vi "Actor Core.vi"(8 "error in":errorcluster, 11 "Pulse Controller in":refnum<class "Pulse Controller.lvclass">) -> (0 "error out":errorcluster, 3 "Actor out":refnum<class "Actor.lvclass">)   [LabVIEW 2016, in "Pulse Controller.lvclass"]
doc: "(<B>Filename</B>: Actor Framework.lvlib:Actor.lvclass:Actor Core.vi)\n\nReceives messages to the actor, reacts to them, and initiates any error handling that may shut the actor down.\n\nDescendant classes may override this VI to append parallel tasks for the actor to complete while it handles messages. Overrides use the Call Parent Method node."
uses:
  Pulse Controller.lvclass
  C:/github/LabActor/Template Module/Template Module.lvclass
  C:/Program Files/National Instruments/LabVIEW 2016/vi.lib/ActorFramework/Actor/Actor.lvclass
  <vilib>/ActorFramework/Actor/Actor.lvclass
  Pulse Controller Configuration.ctl
  Template Module/Template Module.lvclass/Template Module.ctl
  <vilib>/ActorFramework/Actor/Actor.lvclass/Actor.ctl
  <vilib>/ActorFramework/Message Enqueuer/Message Enqueuer.lvclass/Message Enqueuer.ctl
  Template Module/Read stop event.vi
  <vilib>/ActorFramework/Message Enqueuer/Init from Existing Queue.vi
  <vilib>/ActorFramework/Message Enqueuer/Enqueue.vi
  Worker Messages/Trigger Msg/Trigger Msg.lvclass
  C:/Program Files/National Instruments/LabVIEW 2016/vi.lib/ActorFramework/Message/Message.lvclass
  <vilib>/ActorFramework/Message Priority Queue/Priority Enqueue.vi
  Process Controller/Process Controller.lvclass
  <vilib>/ActorFramework/Message Enqueuer/Message Enqueuer.lvclass
panel:
  in  "Trigger":bool
  in  "Configuration":T1={"Pre-trigger duration"=-1.0, "Post-trigger duration"=-1.0, "Open plot after pulse"=TRUE} {"Pre-trigger duration" format="%#_6p"; "Post-trigger duration" format="%#_6p"}
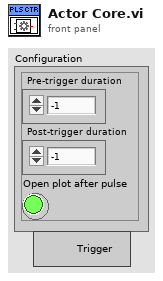
[diagram p1: front panel]
types:
  T1 = typedef "Pulse Controller Configuration.ctl" = cluster{"Pre-trigger duration":dbl, "Post-trigger duration":dbl, "Open plot after pulse":bool}
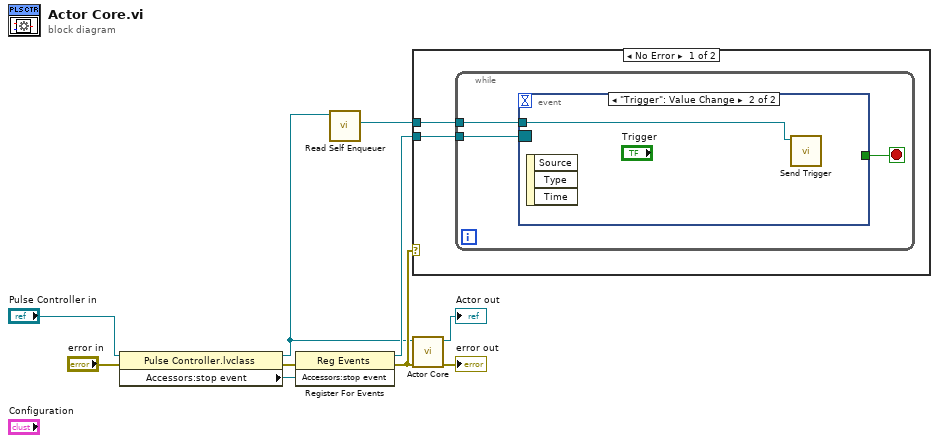
[diagram p0: block diagram]
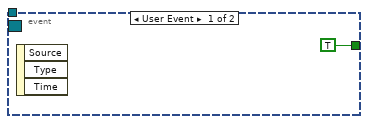
[diagram p2: hidden frame]
diagram:
  n1 = property class="Pulse Controller.lvclass"(reference="Pulse Controller in", error in="error in") -> (reference out=w1:refnum<class "Pulse Controller.lvclass">, error out=w8:errorcluster, "Accessors:stop event"=w7:refnum<user-event>)
  n2 = register-events(error in=w8, w7) -> (reference out=w5:refnum<event-registration>, error out=w2:errorcluster)  [unwired: 1 in]
  n3 = call <vilib>:"Read Self Enqueuer.vi"("Actor"=w1) -> ("Self Enqueuer"=w6:refnum<class "Message Enqueuer.lvclass">)  [unwired: 10 in]
  n4 = case shown="No Error" w2 {
    tunnel: w5 -> [w12 _]
    tunnel: w6 -> [w11 _]
    frame No Error {
      n5 = while {
        tunnel: w12 -> [w15]
        tunnel: w11 -> [w13]
        stop <- w14 stop-if-true
        n6 = event shown="[1] \"Trigger\": Value Change" {
          selector: w15 -> [_ _]
          dyn-events: _ -> [_ _]
          timeout: _ -> [_ _]
          tunnel: [TRUE _] -> w14
          tunnel: w13 -> [_ w17]
          event User Event {
            n7 = event-data() -> ()  [unwired: 1 in, 3 out]
          }
          event "Trigger": Value Change {
            n8 = event-data() -> ()  [unwired: 1 in, 3 out]
            n9 = call "Send Trigger.vi"("Message Enqueuer"=w17) -> ()  [unwired: 9 in, 2 out]
          }
        }
      }
    }
    frame Error {
    }
  }
  n10 = call-parent "Actor Core.vi"("error in"=w2, "Measure Object in"=w1) -> ("error out"=→"error out":errorcluster, "Actor out"=→"Actor out":refnum<class "Actor.lvclass">)  [unwired: 8 in]
